vi "Acq Fetch Waveform (I16 Data Ref).vi"(0 "session in":refnum<class "Digitizer Control.lvclass">, 2 "elements to read":u32, 5 "error in (no error)":errorcluster, 7 "timeout (ms)":i32=5000, 8 "channel index":i32, 9 "clear time out error? (F)":bool) -> (13 "timed out?":bool, 14 "session out":refnum<class "Digitizer Control.lvclass">, 15 "sample data":refnum<data-value>, 16 "elements in region":u32, 17 "elements remaining":u32, 19 "error out":errorcluster)   [LabVIEW 2021, in "Digitizer Control.lvclass"]
doc: "This VI returns a reference to the host DMA buffer part containing the requested amount of acquired sample data as an array of I16s. Use the <B>Acq Configure Channel.vi</B> to configure the channel parameters, the <B>Acq Configure Transfer.vi</B> to configure the waveform transfer, and the <B>Acq Configure Start Trigger.vi</B> to configure the start trigger, then use the <B>Acq Initiate.vi</B> to initiate the acquisition. After the acquisition is initiated, use this VI to fetch the acquired sample data. Use the <B>Acq Get Status.vi</B> to check the acquisition status and the <B>Acq Stop.vi</B> to stop an acquisition.\n\nInputs:\n\n<B>session in</B>: The device session.\n\n<B>channel index</B>: The index of the channel to read.\n\n<B>elements to read</B>: The desired number of I16 elements the referenced array should contain. The actual number of elements is returned on the <B>elements in region</B> output.\n\n<B>timeout</B>: The maximum amount of time, in milliseconds, this VI is allowed to wait for the requested number of elements to become available.\n\n<B>clear time out error?</B>: If this input is true, then the <B>error out</B> output does not return the time out error.\n\nOutputs:\n\n<B>session out</B>: The device session passed on the <B>session in</B> input.\n\n<B>sample data</B>: Reference to an array of I16s containing the acquired sample data. The samples are using fixed point representation: the size of a sample is <B>sample size (bits)</B> bits. The bits of the samples are placed in the I16 elements with LSB first bit packing. To convert the returned I16 array to samples scaled to Volts: unpack the samples then multiply the samples by <B>sample scale factor</B> * 2^-( <B>sample size (bits)</B> ), where <B>sample scale factor</B> is returned by the <B>Acq Configure Channel.vi</B>, while <B>sample size (bits)</B> is returned by the <B>Acq Configure Transfer.vi</B>. The size of the array referenced by this output is returned on the <B>elements in region</B> output. NOTE: The returned data value reference must be deleted after it is no longer needed.\n\n<B>elements in region</B>: The number of I16 elements available in the array referenced by the <B>sample data</B> output.\n\n<B>elements remaining</B>: The number of additional elements remaining in the host DMA buffer that are available for reading.\n\n<B>timed out?</B>: A true on this output indicates that the fetch operation timed out.\n\nNotes:\n\nDo not mix the different Acq Fetch Waveform VIs. Once this VI is called on a channel, use only this VI to fetch the acquired samples on that channel. If you want to use another fetch VI, then it is recommended to reconfigure the transfer first using the <B>Acq Configure Transfer.vi</B>."
uses:
  Digitizer Control.lvclass
  Digitizer Control.lvclass/Digitizer Control.ctl
  <vilib>/Utility/error.llb/Error Cluster From Error Code.vi
  <vilib>/rvi/errors/niLvFpgaAdjustHostInterfaceError.vi
  <vilib>/rvi/interface/nirviMethod/nirviMethod.xnode
  <vilib>/ErrorRing/Error Ring.xnode
  <vilib>/FPGAPlugInAG/Dynamic/niLvFpga_AcquireReadRegionFifo_Dynamic.vi
  <vilib>/rvi/errors/niLvFpgaMergeErrorWithErrorCode.vi
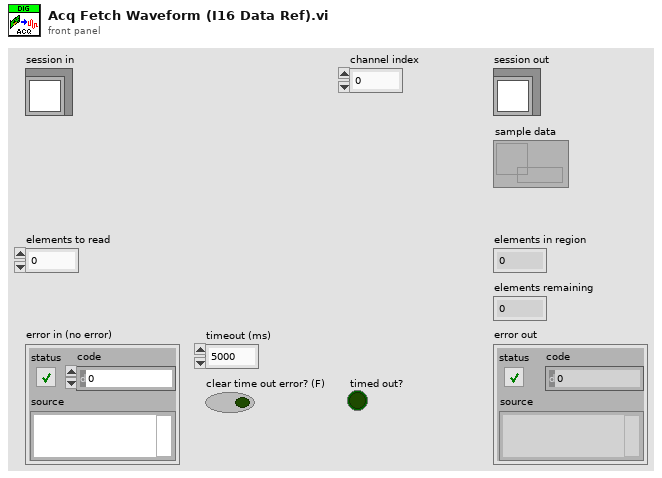
[diagram p1: front panel]
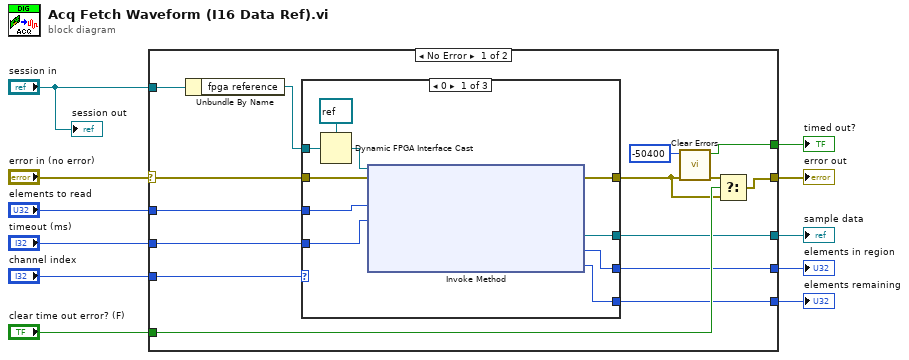
[diagram p0: block diagram]
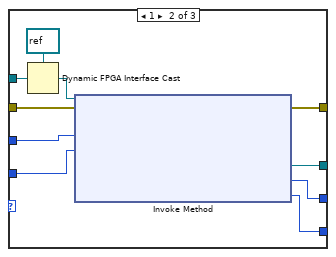
[diagram p2: hidden frame]
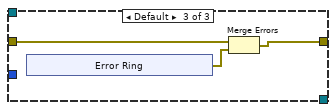
[diagram p3: hidden frame]
diagram:
  n1 = case shown="No Error" "error in (no error)" {
    selector: "error in (no error)" -> [w19 w55]
    tunnel: "elements to read" -> [w23 _]
    tunnel: [w14 w55] -> w4
    tunnel: "timeout (ms)" -> [w25 _]
    tunnel: "session in" -> [w24 _]
    tunnel: [w21 _] -> w8
    tunnel: [w22 _] -> w6
    tunnel: [w20 _] -> w5
    tunnel: "clear time out error? (F)" -> [w26 _]
    tunnel: [w13 _] -> w2
    tunnel: "channel index" -> [w12 _]
    frame No Error {
      n2 = Unbundle By Name(w24) -> ("fpga reference"=w18:refnum<k20>)
      n3 = case shown="0" w12 {
        tunnel: w25 -> [w36 w46 _]
        tunnel: w23 -> [w33 w43 _]
        tunnel: [w32 w42 _] -> w22
        tunnel: [w31 w41 _] -> w21
        tunnel: [w30 w40 _] -> w20
        tunnel: w19 -> [w29 w39 w48]
        tunnel: w18 -> [w28 w38 _]
        tunnel: [w27 w37 w47] -> w15
        frame 0 {
          n4 = Dynamic FPGA Interface Cast(Session In=refnum<k20> refnum ("Type"), Type=w28) -> (Session Out=w35:refnum<k20>)
          n5 = xnode "Invoke Method"("FPGA VI Reference In"=w35, "error in"=w29, "Number of Elements"=w33, "Timeout (ms)"=w36) -> ("error out"=w27:errorcluster, "Read Region Reference"=w32:refnum<data-value>, "Elements In Region"=w30:u32, "Elements Remaining"=w31:u32)  [unwired: 1 out]
        }
        frame 1 {
          n6 = Dynamic FPGA Interface Cast(Session In=refnum<k20> refnum ("Type"), Type=w38) -> (Session Out=w45:refnum<k20>)
          n7 = xnode "Invoke Method"("FPGA VI Reference In"=w45, "error in"=w39, "Number of Elements"=w43, "Timeout (ms)"=w46) -> ("error out"=w37:errorcluster, "Read Region Reference"=w42:refnum<data-value>, "Elements In Region"=w40:u32, "Elements Remaining"=w41:u32)  [unwired: 1 out]
        }
        frame Default {
          n8 = xnode "Error Ring"() -> ("error out"=w49:errorcluster)
          n9 = Merge Errors(w48, w49) -> (w47:errorcluster)
        }
      }
      n10 = call <vilib>:"Clear Errors.vi"("error in (no error)"=w15, "specific error code to clear (0: all)"=-50400) -> ("error out"=w16:errorcluster, "specific error cleared?"=w13:bool)  [unwired: 4 in]
      n11 = Select(t=w16, s=w26, f=w15) -> (s? t:f=w14:errorcluster)
    }
    frame Error {
    }
  }
  "elements remaining" <- w8
  "sample data" <- w6
  "elements in region" <- w5
  "error out" <- w4
  "timed out?" <- w2
  "session out" <- "session in"
